vi "Draw_graph_background.vi"(4 "Y Scale.Range":T2, 5 "ImgRA":dbl, 6 "X Scale.Range":T2, 7 "ImgDEC":dbl, 8 "Field Astrometry":T1, 9 "New Width":i32=300, 10 "New Height":i32=300, 11 "path":path) -> (0 "ImgData":sgl[][](array[numeric]), 1 "Astrometry":T1, 2 "error out":errorcluster, 3 "Images":picture)   [LabVIEW 2019]
uses:
  <vilib>/Utility/miscctls.llb/LVRangeTypeDef.ctl
  gfitsio/gfitsio-read-image-subset-sgl-2d.vi
  gfitsio/gfitsio.lvlib
panel:
  out "Intensity Graph":sgl[][](graph)
  out "header":string[](array[string])
  out "naxis2":i32
  out "naxis1":i32
  out "fpixel (1,1)":cluster{"X":i32, "Y":i32}={"X"=1, "Y"=1}
  out "lpixel (-1,-1: rest)":cluster{"X":i32, "Y":i32}={"X"=-1, "Y"=-1}
  # "(0,0)"
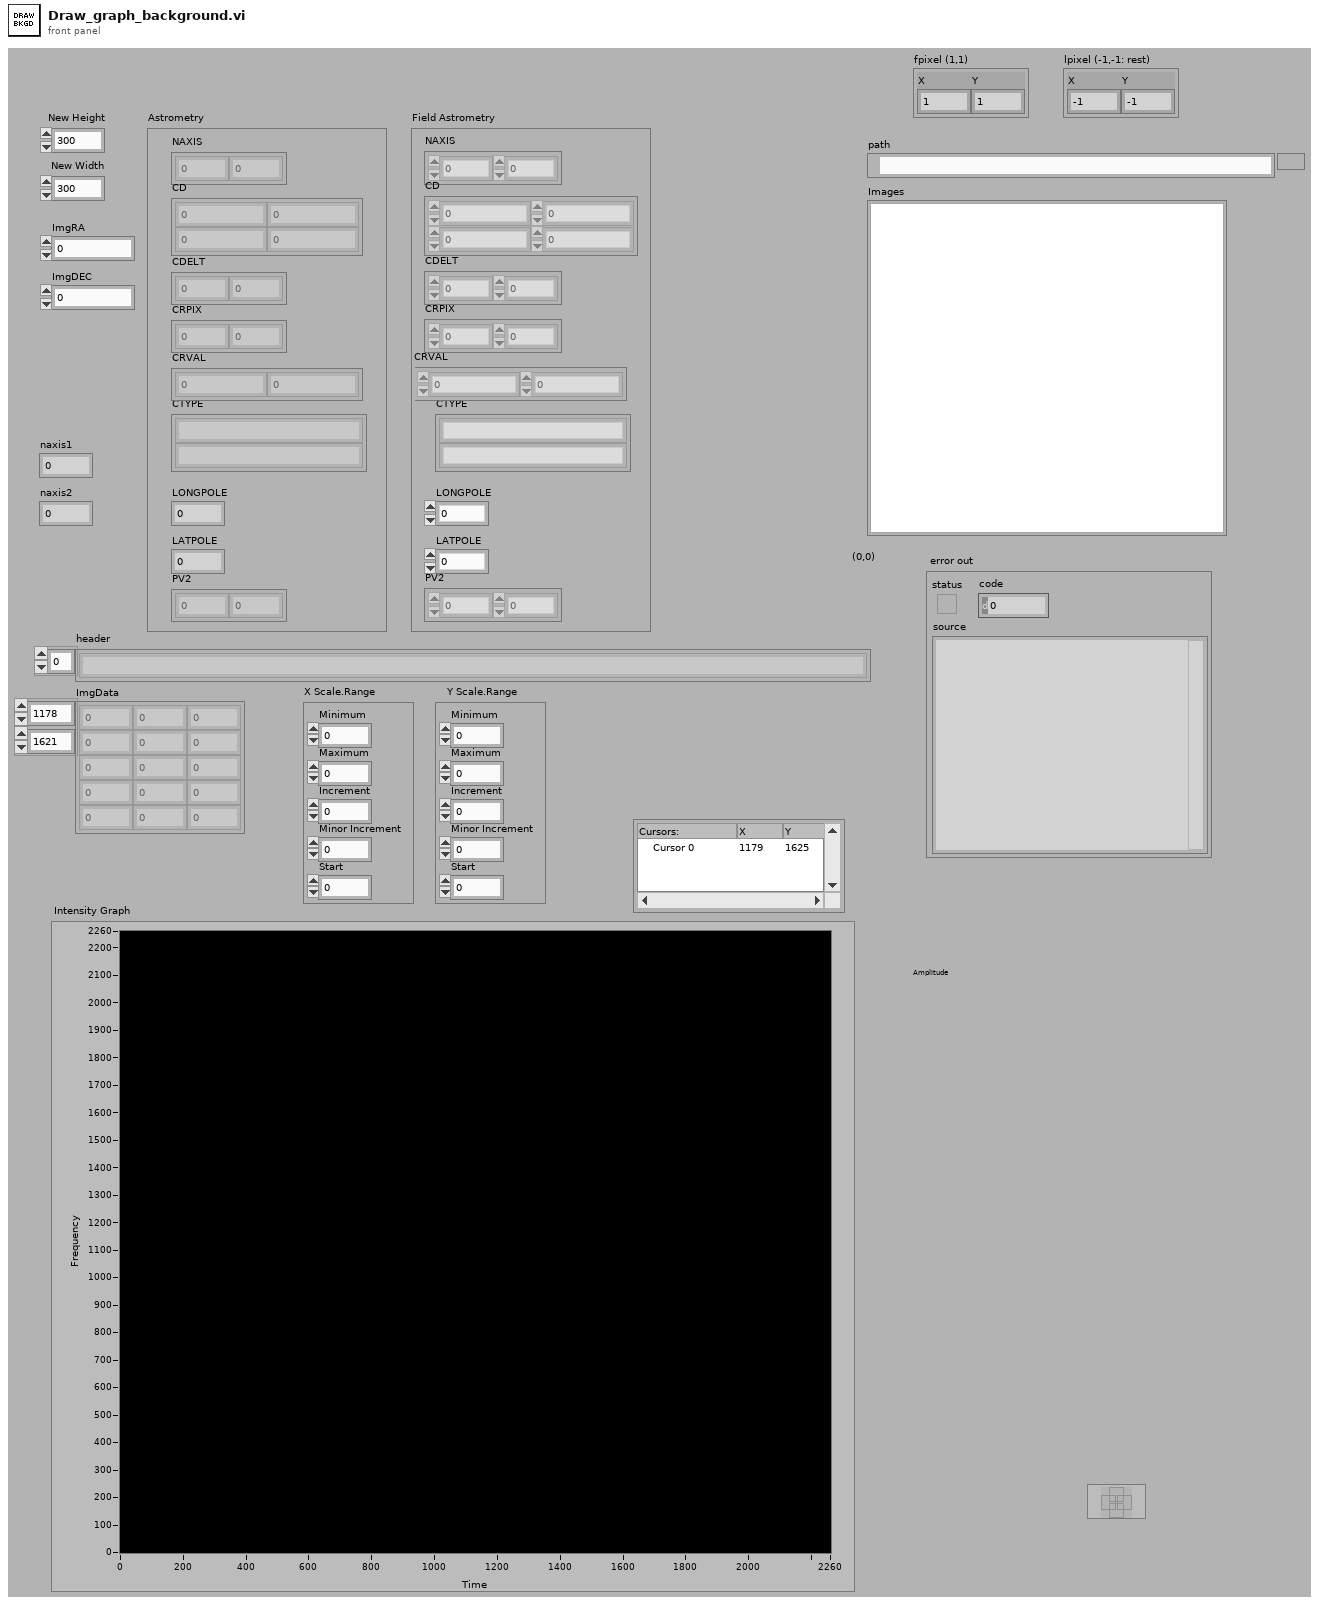
[diagram p1: front panel]
types:
  T1 = cluster{"NAXIS":dbl[], "CD":dbl[][], "CDELT":dbl[], "CRPIX":dbl[], "CTYPE":string[], "CRVAL":dbl[], "LONGPOLE":dbl, "LATPOLE":dbl, "PV2":dbl[]}
  T2 = typedef "LVRangeTypeDef.ctl" = cluster{"Minimum":dbl, "Maximum":dbl, "Increment":dbl, "Minor Increment":dbl, "Start":dbl}
  T3 = typedef "gfitsio.lvlib/gfitsio-refnum.ctl" = refnum<k1>
  T4 = typedef "imagedata.ctl" = cluster{"image type":i32, "image depth":i32, "image":u8[], "mask":u8[], "colors":u32[], "Rectangle":cluster{"left":i16, "top":i16, "right":i16, "bottom":i16}}
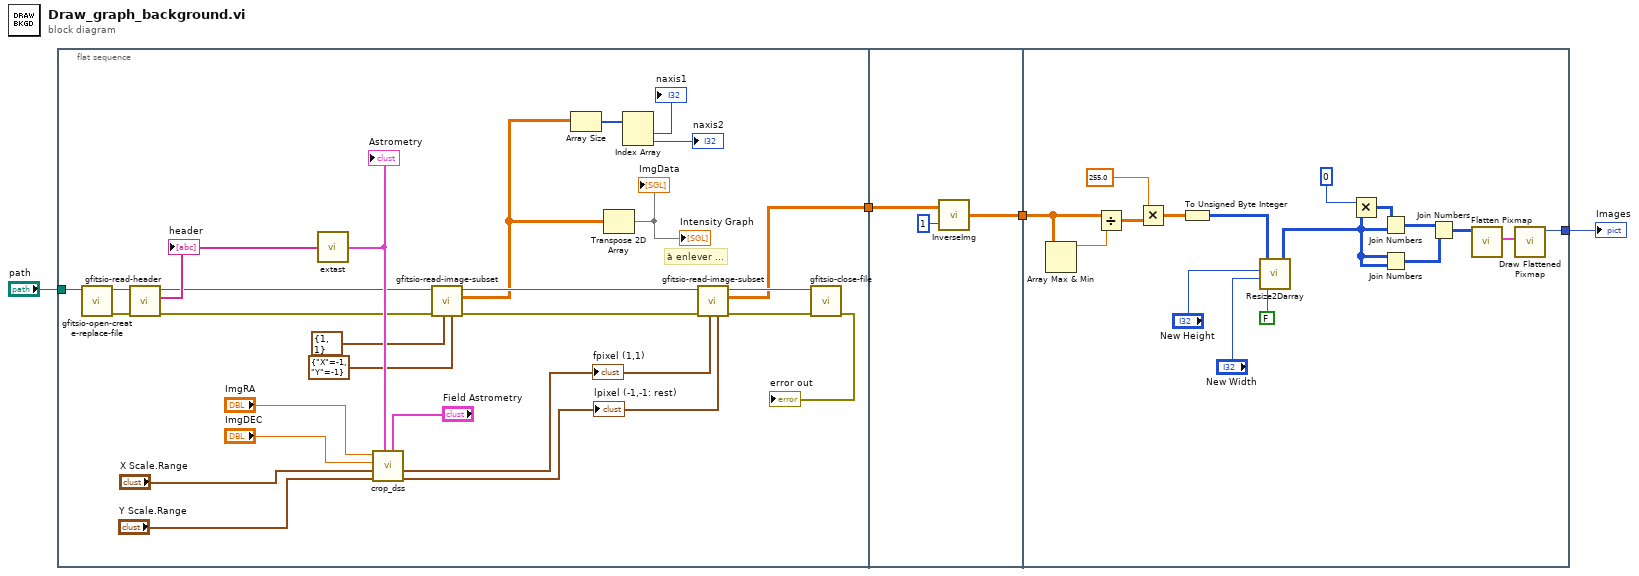
[diagram p0: block diagram]
diagram:
  n1 = flat-sequence {
    tunnel: [w22] -> w1
    tunnel: "path" -> [w26]
    tunnel: [w33] -> w2
    tunnel: w1 -> [w32]
    tunnel: [w47] -> w4
    tunnel: w2 -> [w35]
    frame #0 {
      # "à enlever ..."
      n2 = call "gfitsio-open-create-replace-file.vi"("file path (dialog if empty)"=w26) -> ("error out"=w28:errorcluster, "gfits refnum"=w27:T3)  [unwired: 8 in, 1 out]
      n3 = call "gfitsio-read-header.vi"("error in (no error)"=w28, "gfits refnum"=w27) -> ("error out"=w13:errorcluster, "header"=w31:string[], "dup gfits refnum"=w14:T3)  [unwired: 7 in]
      "header" <- w31
      n4 = call "extast.vi"("header"=w31) -> ("Astrometry"=w21:T1)  [unwired: 14 in]
      "Astrometry" <- w21
      n5 = call "crop_dss.vi"("Field_Astrom"="Field Astrometry", "Img Astrometry"=w21, "Y Scale.Range"="Y Scale.Range", "X Scale.Range"="X Scale.Range", "Img DEC"="ImgDEC", "Img RA"="ImgRA") -> ("lpixel (-1,-1: rest)"=w17:cluster{"X":i32, "Y":i32}, "fpixel (1,1)"=w18:cluster{"X":i32, "Y":i32})  [unwired: 4 in]
      "fpixel (1,1)" <- w18
      "lpixel (-1,-1: rest)" <- w17
      n6 = call-poly "gfitsio-read-image-subset.vi"("lpixel (-1,-1: rest)"=cluster{"X":i32, "Y":i32} {"X"=-1, "Y"=-1}, "fpixel (1,1)"=cluster{"X":i32, "Y":i32} {"X"=1, "Y"=1}, "error in (no error)"=w13, "gfits refnum"=w14) -> ("error out"=w11:errorcluster, "data"=w8:sgl[][], "dup gfits refnum"=w12:T3)  [unwired: 4 in, 1 out]
      n7 = Array Size(array=w8) -> (size(s)=w23:i32[])
      n8 = Transpose 2D Array(2D array=w8) -> (transposed array=→"ImgData" →"Intensity Graph":sgl[][])
      n9 = Index Array(array=w23) -> (element #1=→"naxis1":i32, element #2=→"naxis2":i32)  [unwired: 2 in]
      n10 = call-poly "gfitsio-read-image-subset.vi"("lpixel (-1,-1: rest)"=w17, "fpixel (1,1)"=w18, "error in (no error)"=w11, "gfits refnum"=w12) -> ("error out"=w30:errorcluster, "data"=w22:sgl[][], "dup gfits refnum"=w29:T3)  [unwired: 4 in, 1 out]
      n11 = call "gfitsio-close-file.vi"("error in (no error)"=w30, "gfits refnum"=w29) -> ("error out"=→"error out":errorcluster)  [unwired: 8 in, 1 out]
    }
    frame #1 {
      n12 = call "InverseImg.vi"("MirrorAxis (0=y, 1=x)"=1 ("MirrorAxis"), "Array"=w32) -> ("InvertedImg"=w33:sgl[][])  [unwired: 2 in]
    }
    frame #2 {
      n13 = Array Max & Min(array=w35) -> (max value=w51:sgl)  [unwired: 3 out]
      n14 = Divide(x=w35, y=w51) -> (x/y=w49:sgl[][])
      n15 = Multiply(x=255.0, y=w49) -> (x*y=w39:dbl[][])
      n16 = To Unsigned Byte Integer(number=w39) -> (unsigned 8bit integer=w38:u8[][])
      n17 = call "Resize2Darray.vi"("Maintain Aspect ratio? (T)"=FALSE, "New Width"="New Width", "New Height"="New Height", "2D Array In"=w38) -> ("Resized Array"=w36:u8[][])  [unwired: 3 in]
      n18 = Multiply(x=u8 0, y=w36) -> (x*y=w43:u8[][])
      n19 = Join Numbers(hi=w43, lo=w36) -> ((hi.lo)=w46:u16[][])
      n20 = Join Numbers(hi=w36, lo=w36) -> ((hi.lo)=w45:u16[][])
      n21 = Join Numbers(hi=w46, lo=w45) -> ((hi.lo)=w37:u32[][])
      n22 = call <vilib>:"Flatten Pixmap.vi"("24-bit pixmap"=w37) -> ("image data"=w48:T4)  [unwired: 10 in]
      n23 = call <vilib>:"Draw Flattened Pixmap.vi"("image data"=w48) -> ("new picture"=w47:picture)  [unwired: 8 in]
    }
  }
  "Images" <- w4
